vi "test_CallReserveSessionsWithZeroElementArray_ErrorReturned.vi"(8 "error in":errorcluster) -> (0 "error out":errorcluster, 2 "result":string, 3 "pass":bool)   [LabVIEW 2020, in "MeasurementServerTests.lvlib"]
uses:
  MeasurementServerTests.lvlib
  Runtime/MeasurementLink Measurement Server/Measure Call Context/Measure Call Context.lvclass
  Runtime/MeasurementLink Measurement Server/Helpers/TypeDefs/Pin Map Context.ctl
  Runtime/MeasurementLink Measurement Server/MeasurementLink Measurement Server.lvlib
  <vilib>/gRPC/LabVIEW gRPC Library/Shared/grpcId.ctl
  <vilib>/gRPC/LabVIEW gRPC Library/grpc-lvsupport-release.lvlib
  Runtime/MeasurementLink Measurement Server/IMeasurement Service/IMeasurement Service.lvclass
  Runtime/MeasurementLink Measurement Server/Measurement Plugin Service/Measurement Plugin Service.lvclass
  Runtime/Generated/Measurement Plugin Session Management Client/RPC Messages/nidevice_grpc_Session.ctl
  Runtime/Generated/Measurement Plugin Session Management Client/MeasurementLink Session Management Client.lvlib
  Runtime/Generated/Measurement Plugin Session Management Client/RPC Messages/ni_measurementlink_sessionmanagement_v1_ChannelMapping.ctl
  Runtime/Generated/Measurement Plugin Session Management Client/RPC Messages/ni_measurementlink_sessionmanagement_v1_SessionInformation.ctl
  Runtime/MeasurementLink Measurement Server/Measure Call Context/Data.ctl
  Runtime/MeasurementLink Measurement Server/Helpers/Error Strings Global Internal.vi
  Runtime/MeasurementLink Measurement Server/Measure Call Context/Reserve Sessions - NPin.vi
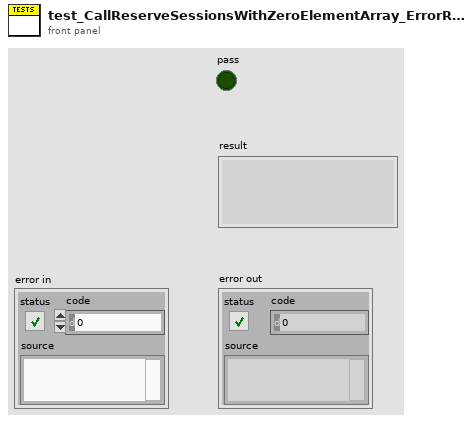
[diagram p1: front panel]
types:
  T1 = typedef "MeasurementLink Measurement Server.lvlib/Measure Call Context.lvclass/Data.ctl" = cluster{"pin map context":T2, "gRPC ID":T3, "measurement service":refnum<class "IMeasurement Service.lvclass">, "measurement plugin service":refnum<class "Measurement Plugin Service.lvclass">, "reserved session infos":set{T4}}
  T2 = typedef "MeasurementLink Measurement Server.lvlib/Pin Map Context.ctl" = cluster{"pin map id":string, "sites":i32[]}
  T3 = typedef "grpc-lvsupport-release.lvlib/grpcId.ctl" = u64
  T4 = typedef "MeasurementLink Session Management Client.lvlib/ni_measurementlink_sessionmanagement_v1_SessionInformation.ctl" = cluster{"session":T5, "resource_name":string, "channel_list":string, "instrument_type_id":string, "session_exists":bool, "channel_mappings":T6[]}
  T5 = typedef "MeasurementLink Session Management Client.lvlib/nidevice_grpc_Session.ctl" = cluster{"name":string}
  T6 = typedef "MeasurementLink Session Management Client.lvlib/ni_measurementlink_sessionmanagement_v1_ChannelMapping.ctl" = cluster{"pin_or_relay_name":string, "site":i32, "channel":string, "multiplexer_resource_name":string, "multiplexer_route":string}
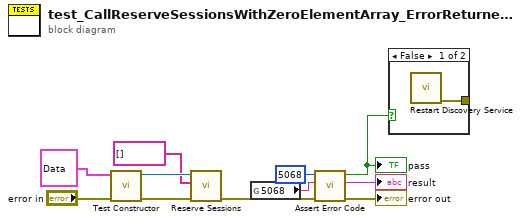
[diagram p0: block diagram]
diagram:
  n1 = call "Test Constructor.vi"("error in"="error in", "data"=T1 {"pin map context"={"pin map id"="", "sites"=[]}, "gRPC ID"=0, "measurement service"=refnum, "measurement plugin service"=refnum, "reserved session infos"={}}) -> ("error out"=w11:errorcluster, "measure call context out"=w10:refnum<class "Measure Call Context.lvclass">)  [unwired: 8 in]
  n2 = call-poly "Reserve Sessions.vi"("error in"=w11, "pin or relay names"=string[] [], "measurement context in"=w10) -> ("error out"=w9:errorcluster)  [unwired: 6 in, 2 out]
  n3 = global read "Error Strings Global Internal.vi" "5068"() -> (w6:string)
  n4 = call "Assert Error Code.vi"("error in"=w9, "expected error description"=w6, "expected error code"=5068) -> ("error out"=→"error out":errorcluster, "details"=→"result":string, "error code match?"=w2:bool)  [unwired: 6 in]
  "pass" <- w2
  n5 = case shown="False" w2 {
    tunnel: [w12 _] -> _
    frame False {
      n6 = call "Restart Discovery Service.vi"() -> ("error out"=w12:errorcluster)  [unwired: 11 in]
    }
    frame True {
    }
  }
